vi "CM_split string.vi"(8 "error in (no error)":errorcluster, 9 "search string":string, 10 "String":string) -> (0 "error out":errorcluster, 2 "strings array":string[](array[string]))   [LabVIEW 2018]
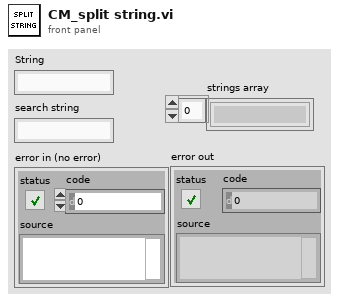
[diagram p1: front panel]
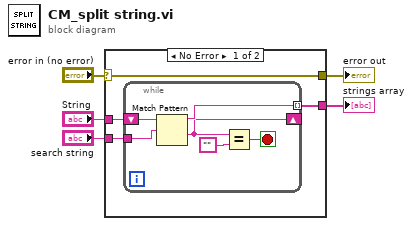
[diagram p0: block diagram]
diagram:
  n1 = case shown="No Error" "error in (no error)" {
    selector: "error in (no error)" -> [w9 w16]
    tunnel: [w9 w16] -> w4
    tunnel: "search string" -> [w8 _]
    tunnel: "String" -> [w7 _]
    tunnel: [w6 _] -> w1
    frame No Error {
      n2 = while {
        shift-right: [w10] -> _
        shift-left: w7 -> [w13]
        tunnel: w8 -> [w12]
        tunnel: [w11] -> w6 mode=indexing
        stop <- w14 stop-if-true
        n3 = Match Pattern(string=w13, regular expression=w12) -> (before substring=w11:string, after substring=w10:string)  [unwired: 1 in, 2 out]
        n4 = Equal?(x=w10, y="") -> (x = y?=w14:bool)
      }
    }
    frame Error {
    }
  }
  "error out" <- w4
  "strings array" <- w1
